vi "Calculate Temperature Change.vi"(7 "Ramp Rate deg C/s":dbl, 8 "Shutdown":bool, 9 "Time Interval (s)":dbl, 10 "Actual Temperature in deg C":dbl, 11 "Required Temperature deg C":dbl) -> (3 "Actual Temperature out":dbl)   [LabVIEW 2018, in "Thermal Chamber Response Simulator.lvlib"]
uses:
  Thermal Chamber Response Simulator.lvlib
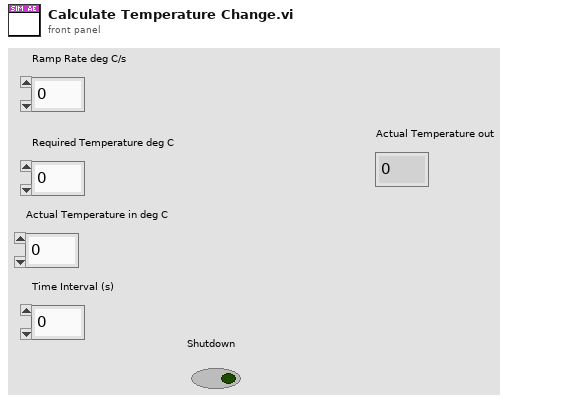
[diagram p1: front panel]
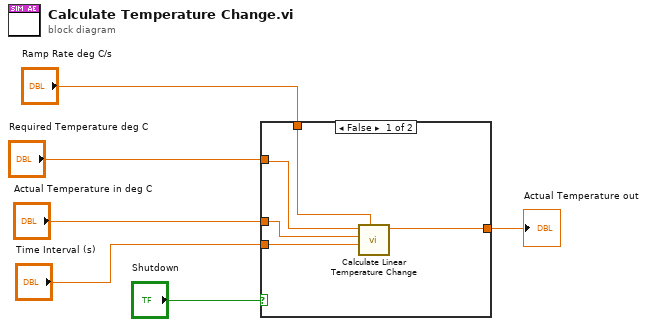
[diagram p0: block diagram]
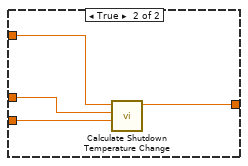
[diagram p2: hidden frame]
diagram:
  n1 = case shown="False" "Shutdown" {
    tunnel: "Required Temperature deg C" -> [w9 w15]
    tunnel: "Actual Temperature in deg C" -> [w10 w14]
    tunnel: "Time Interval (s)" -> [w11 w13]
    tunnel: [w7 w12] -> w2
    tunnel: "Ramp Rate deg C/s" -> [w8 _]
    frame False {
      n2 = call "Calculate Linear Temperature Change.vi"("Ramp Rate deg C/s"=w8, "Time Interval (s)"=w11, "Actual Temperature in"=w10, "Required Temperature deg C"=w9) -> ("Actual Temperature out"=w7:dbl)  [unwired: 7 in]
    }
    frame True {
      n3 = call "Calculate Shutdown Temperature Change.vi"("Interval"=w13, "Actual Temperature In"=w14, "Required Temperature deg C"=w15) -> ("Actual Temperature Out"=w12:dbl)  [unwired: 8 in]
    }
  }
  "Actual Temperature out" <- w2
